vi "Initialise.vi"(11 "Position":refnum<class "Vector 2D.lvclass">) -> (3 "Thrust Dot out":refnum<class "Thrust Dot.lvclass">)   [LabVIEW 2021, in "Thrust Dot.lvclass"]
uses:
  Thrust Dot.lvclass
  Vector 2D/Vector 2D.lvclass
  Thrust Dot.lvclass/Thrust Dot.ctl
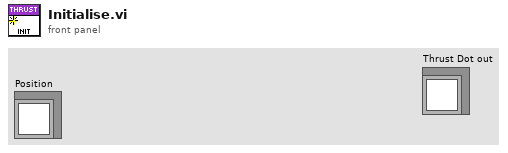
[diagram p1: front panel]
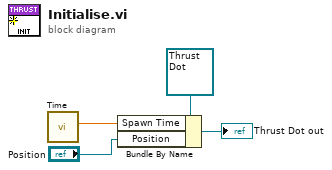
[diagram p0: block diagram]
diagram:
  n1 = call "Time.vi"() -> ("Time [s]"=w1:sgl)  [unwired: 10 in, 1 out]
  n2 = Bundle By Name(cluster=refnum<class "Thrust Dot.lvclass"> refnum ("Thrust Dot in"), "Spawn Time"=w1, "Position"="Position") -> (→"Thrust Dot out":refnum<class "Thrust Dot.lvclass">)
